vi "Prax12.1.vi"() -> ()   [LabVIEW 2020]
panel:
  in  "Path":path
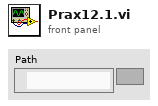
[diagram p1: front panel]
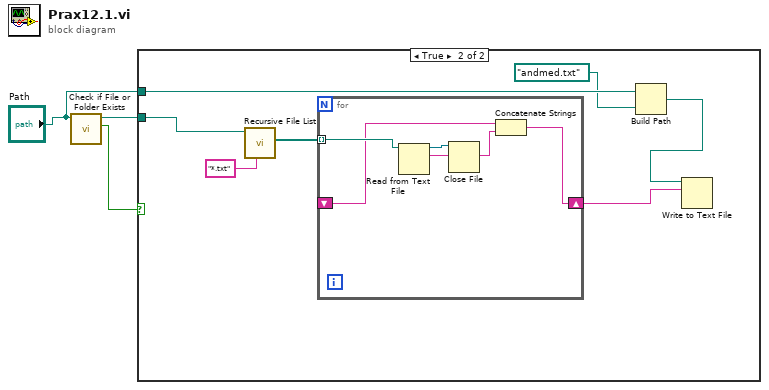
[diagram p0: block diagram]
diagram:
  n1 = call <vilib>:"Check if File or Folder Exists.vi"("path"="Path") -> ("file or folder exists?"=w3:bool, "dup path"=w2:path)  [unwired: 8 in, 1 out]
  n2 = case shown="True" w3 {
    tunnel: w2 -> [_ w10]
    tunnel: "Path" -> [_ w6]
    frame False {
    }
    frame True {
      n3 = call <vilib>:"Recursive File List.vi"("pattern"="*.txt", "Folder Path"=w10) -> ("All Files in Dir"=w8:path[])  [unwired: 5 in, 4 out]
      n4 = for {
        tunnel: w8 -> [w15] mode=indexing
        shift-right: [w12] -> w7
        shift-left: _ -> [w14]
        n5 = Read from Text File(file (use dialog)=w15) -> (refnum out=w11:refnum<file>, text=w13:string)  [unwired: 3 in, 2 out]
        n6 = Close File(refnum=w11) -> ()  [unwired: 1 in, 2 out]
        n7 = Concatenate Strings(w14, w13) -> (w12:string)
      }
      n8 = Build Path(base path=w6, name or relative path=path "andmed.txt") -> (appended path=w4:path)
      n9 = Write to Text File(file (use dialog)=w4, text=w7) -> ()  [unwired: 2 in, 3 out]
    }
  }
